vi "Part 2.vi"(11 "Input":string) -> (3 "Output":i64)   [LabVIEW 2021]
uses:
  e083bf95-9e23-4fbb-9388-5321f51aaacc.vi
  <vilib>/Comparison/Less/Less Functor/Less Functor.lvclass
panel:
  out "array":string[](array[string])
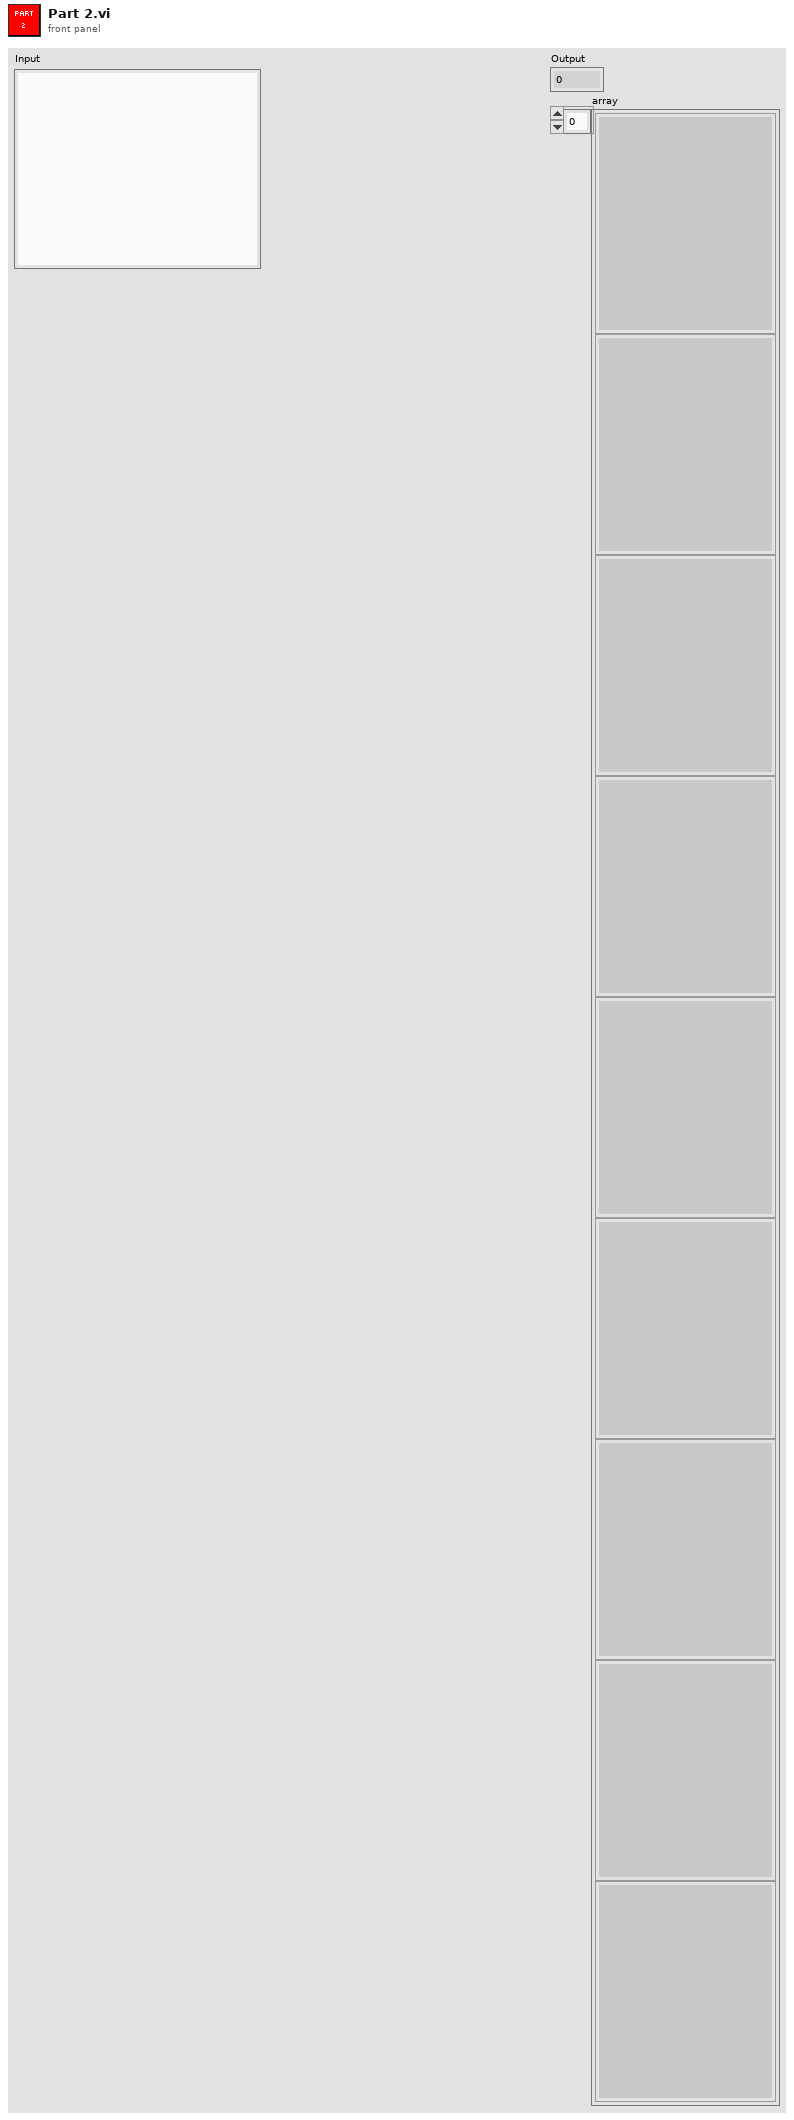
[diagram p1: front panel]
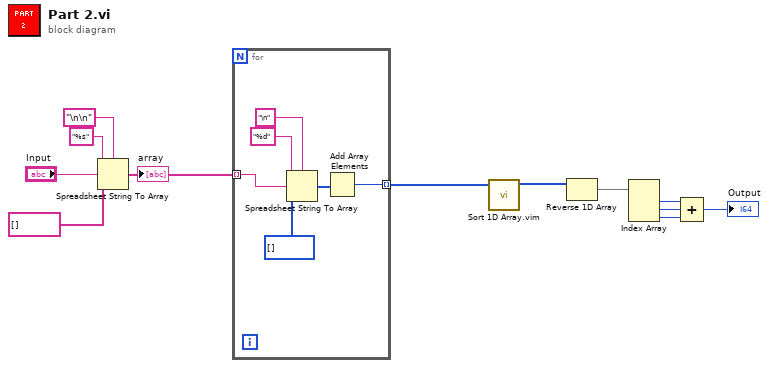
[diagram p0: block diagram]
diagram:
  n1 = Spreadsheet String To Array(delimiter (Tab)="\n\n", format string="%s", spreadsheet string="Input", array type (2D Dbl)=string[] []) -> (array=w8:string[])
  "array" <- w8
  n2 = for {
    tunnel: w8 -> [w16] mode=indexing
    tunnel: [w13] -> w7 mode=indexing
    n3 = Spreadsheet String To Array(delimiter (Tab)="\n", format string="%d", spreadsheet string=w16, array type (2D Dbl)=i64[] []) -> (array=w14:i64[])
    n4 = Add Array Elements(numeric array=w14) -> (sum=w13:i64)
  }
  n5 = call "Sort 1D Array.vim"("unsorted array"=w7) -> ("sorted array"=w6:i64[])  [unwired: 10 in]
  n6 = Reverse 1D Array(array=w6) -> (reversed array=w5:i64[])
  n7 = Index Array(array=w5) -> (element #1=w3:i64, element #2=w4:i64, element #3=w2:i64)  [unwired: 3 in]
  n8 = Compound Arithmetic op=ADD(w3, w4, w2) -> (→"Output":i64)
